vi "Assign 1 EXOR AND EXNOR using NAND GATES.vi"() -> ()   [LabVIEW 2018]
panel:
  out "XNOR GATE USING NAND GATE":bool
  in  "D":bool
  in  "C":bool
  out "XOR GATE USING NAND GATE":bool
  in  "B":bool
  in  "A":bool
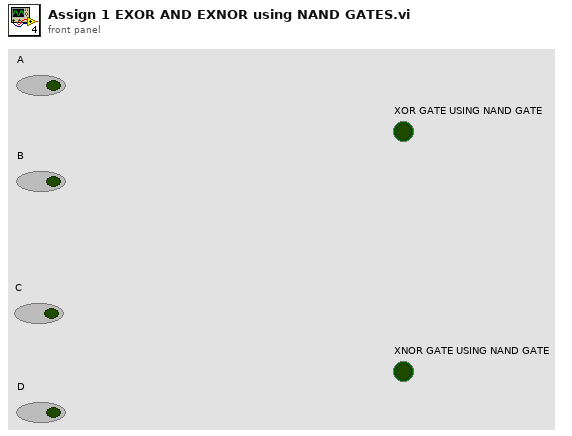
[diagram p1: front panel]
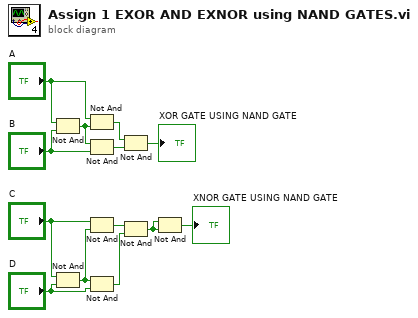
[diagram p0: block diagram]
diagram:
  n1 = Not And(1:"B", 2:"A") -> (0:w11:bool)
  n2 = Not And(1:"D", 2:"C") -> (0:w3:bool)
  n3 = Not And(1:w11, 2:"A") -> (0:w10:bool)
  n4 = Not And(1:"B", 2:w11) -> (0:w9:bool)
  n5 = Not And(1:w3, 2:"C") -> (0:w7:bool)
  n6 = Not And(1:"D", 2:w3) -> (0:w6:bool)
  n7 = Not And(1:w9, 2:w10) -> (0:→"XOR GATE USING NAND GATE":bool)
  n8 = Not And(1:w6, 2:w7) -> (0:w5:bool)
  n9 = Not And(1:w5, 2:w5) -> (0:→"XNOR GATE USING NAND GATE":bool)
